vi "MGI Close Modal Windows.vi"() -> (0 "error out":errorcluster)   [LabVIEW 2020]
doc: "This VI closes any open Modal Windows when called from the LabVIEW development environment. When called from a built executable, it does nothing.\nThis VI is useful to avoid locking up LabVIEW when a top level VI is run while a non-running Modal subVI is open.\n\nAuthored by Stephen Moore\nsupport@mooregoodideas.com\nwww.mooregoodideas.com\n\nCopyright (c) 2010, Moore Good Ideas, Inc.\n\nAll rights reserved.\n\nRedistribution and use in source and binary forms, with or without modification, are permitted provided that the following conditions are met:\n\n * Redistributions of source code must retain the above copyright notice, this list of conditions and the following disclaimer.\n * Redistributions in binary form must reproduce the above copyright notice, this list of conditions and the following disclaimer in the documentation and/or other materials provided with the distribution.\n * Neither the name of Moore Good Ideas, Inc. nor the names of its contributors may be used to endorse or promote products derived from this software without specific prior written permission.\n\nTHIS SOFTWARE IS PROVIDED BY THE COPYRIGHT HOLDERS AND CONTRIBUTORS \"AS IS\" AND ANY EXPRESS OR IMPLIED WARRANTIES, INCLUDING, BUT NOT LIMITED TO, THE IMPLIED WARRANTIES OF MERCHANTABILITY AND FITNESS FOR A PARTICULAR PURPOSE ARE DISCLAIMED. IN NO EVENT SHALL THE COPYRIGHT OWNER OR CONTRIBUTORS BE LIABLE FOR ANY DIRECT, INDIRECT, INCIDENTAL, SPECIAL, EXEMPLARY, OR CONSEQUENTIAL DAMAGES (INCLUDING, BUT NOT LIMITED TO, PROCUREMENT OF SUBSTITUTE GOODS OR SERVICES; LOSS OF USE, DATA, OR PROFITS; OR BUSINESS INTERRUPTION) HOWEVER CAUSED AND ON ANY THEORY OF LIABILITY, WHETHER IN CONTRACT, STRICT LIABILITY, OR TORT (INCLUDING NEGLIGENCE OR OTHERWISE) ARISING IN ANY WAY OUT OF THE USE OF THIS SOFTWARE, EVEN IF ADVISED OF THE POSSIBILITY OF SUCH DAMAGE."
panel:
  in  "error in (no error)":errorcluster
  out "Progress":i32(slide) scale=0.0..5.0
  # "Closing Modal Windows...."
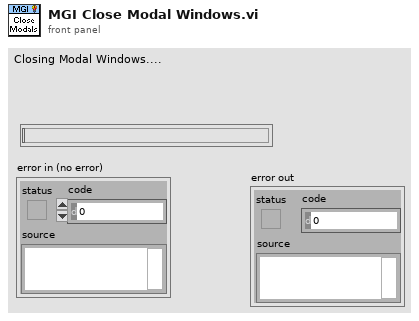
[diagram p1: front panel]
types:
  T1 = enum32{"Invalid", "Standard", "Closed", "Hidden", "Minimized", "Maximized"}
  T2 = enum32{"Invalid", "Default", "Floating", "Floating/Auto-Hide", "Modal"}
  T3 = enum32{"Bad", "Idle", "Run top level", "Running"}
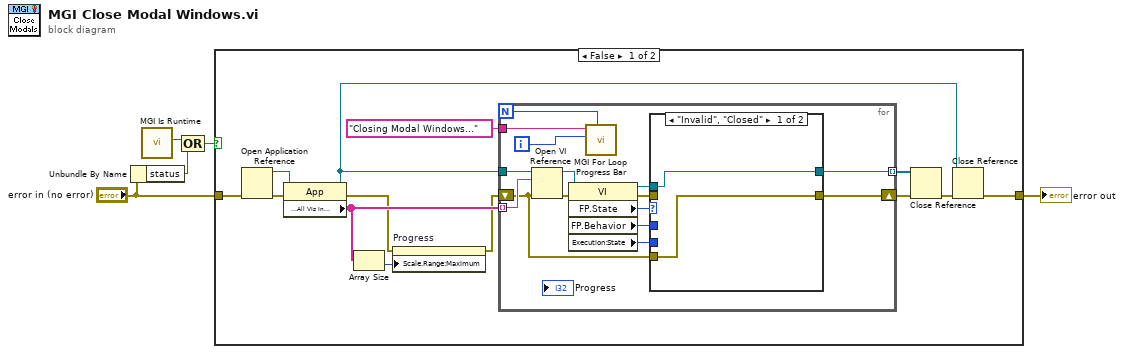
[diagram p0: block diagram]
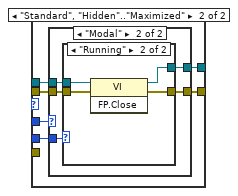
[diagram p2: hidden frame]
diagram:
  n1 = Unbundle By Name("error in (no error)") -> ("status"=w3:bool)
  n2 = call <userlib>:"MGI Is Runtime.vi"() -> ("Run Time System?"=w1:bool)  [unwired: 7 in]
  n3 = Compound Arithmetic op=OR(w1, w3) -> (w2:bool)
  n4 = case shown="False" w2 {
    tunnel: [w13 w55] -> w5
    tunnel: "error in (no error)" -> [w7 w55]
    frame False {
      n5 = Open Application Reference(8:w7) -> (0:w18:errorcluster, 3:w17:refnum<vi>)  [unwired: 3 in]
      n6 = property class="App"(reference=w17, error in=w18) -> (reference out=w15:refnum<vi>, error out=w12:errorcluster, "Application:All VIs In Memory"=w16:string[])
      n7 = Array Size(array=w16) -> (size(s)=w14:i32)
      n8 = property on="Progress" class="Slide (strict)"(error in=w12, "Scale.Range:Maximum"=w14) -> (error out=w11:errorcluster)  [unwired: 1 in, 1 out]
      n9 = for {
        N -> [w19]
        tunnel: w16 -> [w33] mode=indexing
        tunnel: w15 -> [w32]
        tunnel: [w24] -> w10 mode=indexing
        shift-right: [w23] -> w8
        shift-left: w11 -> [w22]
        tunnel: "Closing Modal Windows..." ("Message") -> [w21]
        i -> [w20]
        n10 = Open VI Reference(application reference (local)=w32, vi path=w33, error in (no error)=w22) -> (vi reference=w30:refnum<vi>, error out=w31:errorcluster)  [unwired: 3 in]
        n11 = property class="VI"(reference=w30, error in=w31) -> (reference out=w27:refnum<vi>, error out=w28:errorcluster, "FP.State"=w25:T1, "FP.Behavior"=w26:T2, "Execution:State"=w29:T3)
        n12 = call <userlib>:"MGI For Loop Progress Bar.vi"("Total Iter"=w19, "Current Iter"=w20, "Message"=w21) -> ()  [unwired: 7 in, 2 out]
        n13 = case shown="\"Invalid\", \"Closed\"" w25 {
          tunnel: w29 -> [_ w41]
          tunnel: w28 -> [_ w40]
          tunnel: w27 -> [w35 w39]
          tunnel: [w34 w38] -> w23
          tunnel: [w35 w37] -> w24
          tunnel: w26 -> [_ w36]
          tunnel: w22 -> [w34 _]
          frame "Invalid", "Closed" {
          }
          frame "Standard", "Hidden".."Maximized" {
            n14 = case shown="\"Modal\"" w36 {
              tunnel: w41 -> [_ w48]
              tunnel: w40 -> [w42 w47]
              tunnel: w39 -> [w43 w46]
              tunnel: [w42 w45] -> w38
              tunnel: [w43 w44] -> w37
              frame Default {
              }
              frame "Modal" {
                n15 = case shown="\"Running\"" w48 {
                  tunnel: w47 -> [w49 w54]
                  tunnel: w46 -> [w50 w53]
                  tunnel: [w49 w52] -> w45
                  tunnel: [w50 w51] -> w44
                  frame Default {
                  }
                  frame "Running" {
                    n16 = invoke class="VI" method="FP.Close"(reference=w53, error in=w54) -> (reference out=w51:refnum<vi>, error out=w52:errorcluster)  [unwired: 1 in, 1 out]
                  }
                }
              }
            }
          }
        }
      }
      n17 = Close Reference(reference=w10, error in (no error)=w8) -> (error out=w9:errorcluster)
      n18 = Close Reference(reference=w15, error in (no error)=w9) -> (error out=w13:errorcluster)
    }
    frame True {
      # "If run from an executable nothing will be done"
    }
  }
  "error out" <- w5
